vi "initialize.vi"(0 "HGF_NetworkData":refnum<class "HGF_NetworkVisitor.lvclass">, 3 "initializationData":variant, 5 "error in (no error)":errorcluster, 7 "binaryString":string, 8 "I8 Array":i8[](array[numeric]), 9 "prependSize? (T)":bool, 11 "byteOrder (0:big-endian, network order)":T1(ring)) -> (14 "dup HGF_NetworkData":refnum<class "HGF_NetworkVisitor.lvclass">, 17 "found?":bool, 19 "error out":errorcluster)   [LabVIEW 2014, in "HGF_BaseClasses.lvlib" / "HGF_NetworkVisitor.lvclass"]
doc: "This is a dynamic dispatch VI to be implemented by child classes to initialize their attributes.\n\n<B>Recommendation:</B> Use Variant for initialization data."
uses:
  HGF_NetworkVisitor.lvclass
  HGF_Visitor/HGF_Visitor.lvclass
  HGF_PVSubscriber/HGF_PVSubscriber.lvclass
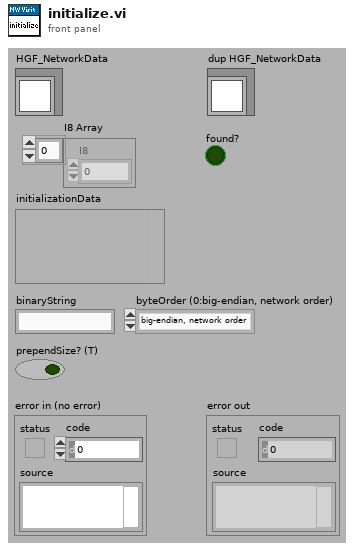
[diagram p1: front panel]
types:
  T1 = enum16{"big-endian, network order", "native, host order", "little-endian"}
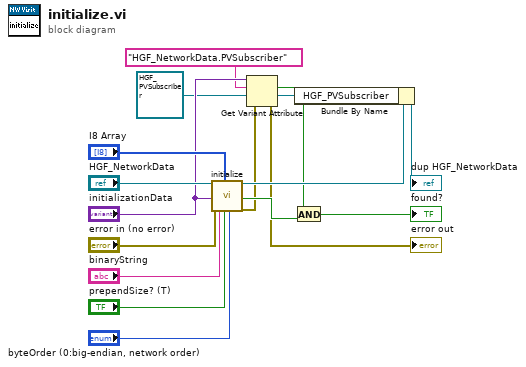
[diagram p0: block diagram]
diagram:
  n1 = call-parent "initialize.vi"("HGF_Visitor"="HGF_NetworkData", "initializationData"="initializationData", "error in (no error)"="error in (no error)", "binaryString"="binaryString", "I8 Array"="I8 Array", "prependSize? (T)"="prependSize? (T)", "byteOrder (0:big-endian, network order)"="byteOrder (0:big-endian, network order)") -> ("dup HGF_Visitor"=w9:refnum<class "HGF_NetworkVisitor.lvclass">, "found?"=w5:bool, "error out"=w3:errorcluster)  [unwired: 10 out]
  n2 = Get Variant Attribute(Variant="initializationData", name="HGF_NetworkData.PVSubscriber", default value (empty Variant)=refnum<class "HGF_PVSubscriber.lvclass"> refnum ("HGF_PVSubscriber"), error in=w3) -> (found=w6:bool, value=w7:refnum<class "HGF_PVSubscriber.lvclass">, error out=→"error out":errorcluster)  [unwired: 1 out]
  n3 = And(x=w6, y=w5) -> (x .and. y?=→"found?":bool)
  n4 = Bundle By Name(cluster=w9, "HGF_PVSubscriber"=w7) -> (→"dup HGF_NetworkData":refnum<class "HGF_NetworkVisitor.lvclass">)
